vi "about get file size.vi"(8 "error in (no error)":errorcluster, 11 "directory path":path) -> (0 "error out":errorcluster, 2 "size":dbl format="%.2f", 3 "subdir_path":path[](array[path]))   [LabVIEW 2011]
doc: "This VI determines the sizes of the files located in the specified directory and also determines the paths of the subdirectories located with the upper level directory."
panel:
  # "This VI determines the sizes of the files located in the specified directory and also \ndetermines the paths of the subdirectories located with the upper level directory."
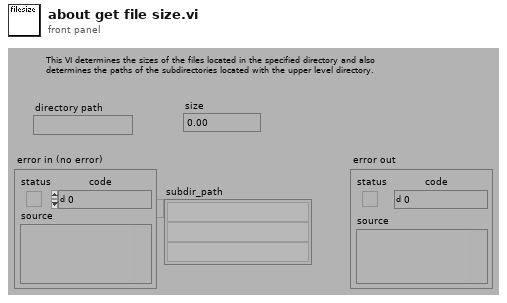
[diagram p1: front panel]
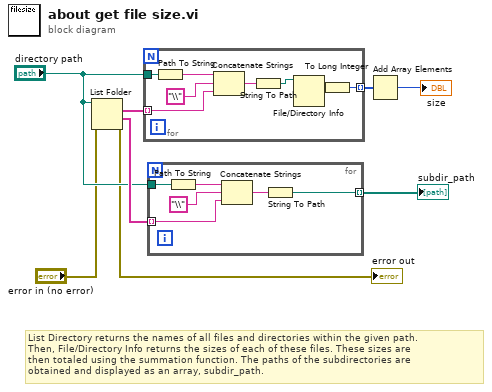
[diagram p0: block diagram]
diagram:
  # "List Directory returns the names of all files and directories within the given path. \nThen, File/Directory Info returns the sizes of each of these files. These sizes are\nthen totaled using the summation function. The paths of the subdirectories are \nobtained and displayed as an array, subdir_path."
  n1 = List Folder(path="directory path", error in="error in (no error)") -> (filenames=w7:string[], folder names=w4:string[], error out=→"error out":errorcluster)  [unwired: 2 in, 1 out]
  n2 = for {
    tunnel: w7 -> [w14] mode=indexing
    tunnel: "directory path" -> [w10]
    tunnel: [w11] -> w8 mode=indexing
    n3 = Path To String(path=w10) -> (string=w16:string)
    n4 = Concatenate Strings(w16, "\\", w14) -> (w13:string)
    n5 = String To Path(string=w13) -> (path=w12:path)
    n6 = File/Directory Info(path=w12) -> (size=w9:i64)  [unwired: 1 in, 6 out]
    n7 = To Long Integer(number=w9) -> (32bit integer=w11:i32)
  }
  n8 = for {
    tunnel: [w19] -> w5 mode=indexing
    tunnel: w4 -> [w18] mode=indexing
    tunnel: "directory path" -> [w17]
    n9 = Path To String(path=w17) -> (string=w22:string)
    n10 = Concatenate Strings(w22, "\\", w18) -> (w20:string)
    n11 = String To Path(string=w20) -> (path=w19:path)
  }
  "subdir_path" <- w5
  n12 = Add Array Elements(numeric array=w8) -> (sum=→"size":i32)
